vi "Master_CAN.vi"(8 "error in":errorcluster) -> (0 "error out":errorcluster)   [LabVIEW 2018]
uses:
  Type_Def/Type_Def Actuator Controls.ctl
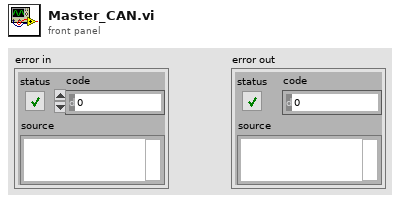
[diagram p1: front panel]
types:
  T1 = typedef "Type_Def Actuator Controls.ctl" = cluster{"Reverse ":bool, "Precharge Ctrl":bool, "Pump Ctrl":bool, "24 VDC Ctr":bool, "Vent Solenoid":bool, "Brake Solenoid":bool, "EMCY  Brake Solenoid":bool, "Digital Out 7B ":bool, "Forward Ctrl":bool, "Contact H1":bool, "Contact L1":bool, "Contact H2":bool, "Contact L2 ":bool, "LED RED":bool, "LED GREEN":bool, " Digital Out 7A":bool}
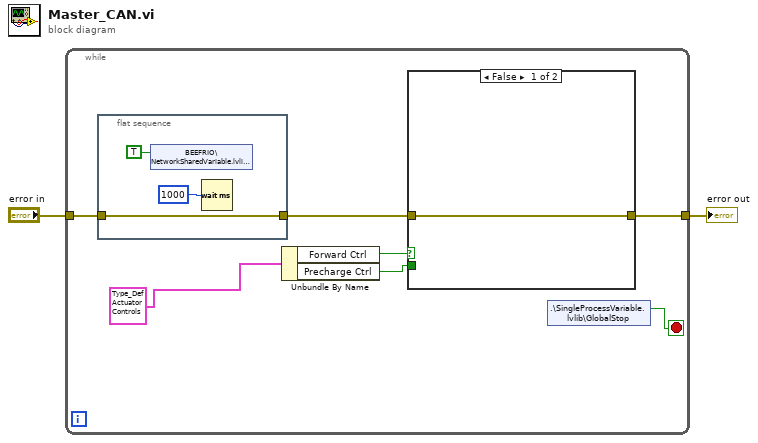
[diagram p0: block diagram]
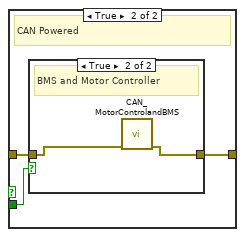
[diagram p2: hidden frame]
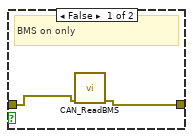
[diagram p3: hidden frame]
diagram:
  n1 = while {
    tunnel: "error in" -> [w8]
    tunnel: [w9] -> w1
    stop <- w6 stop-if-true
    n2 = flat-sequence {
      tunnel: [w19] -> w7
      tunnel: w8 -> [w19]
      frame #0 {
        n3 = shared-variable "BEEFRIO\\NetworkSharedVariable.lvlib\\BMSFreeze"(TRUE ("BMSFreeze")) -> ()  [unwired: 1 in, 1 out]
        n4 = Wait (ms)(milliseconds to wait=u32 1000) -> ()  [unwired: 1 out]
      }
    }
    n5 = Unbundle By Name(T1 {"Reverse "=TRUE, "Precharge Ctrl"=TRUE, "Pump Ctrl"=TRUE, "24 VDC Ctr"=TRUE, "Vent Solenoid"=TRUE, "Brake Solenoid"=TRUE, "EMCY  Brake Solenoid"=TRUE, "Digital Out 7B "=TRUE, "Forward Ctrl"=TRUE, "Contact H1"=TRUE, "Contact L1"=TRUE, "Contact H2"=TRUE, "Contact L2 "=TRUE, "LED RED"=TRUE, "LED GREEN"=TRUE, " Digital Out 7A"=TRUE} ("input cluster")) -> ("Forward Ctrl"=w5:bool, "Precharge Ctrl"=w4:bool)
    n6 = case shown="False" w5 {
      tunnel: [w10 w13] -> w9
      tunnel: w7 -> [w10 w12]
      tunnel: w4 -> [_ w11]
      frame False {
      }
      frame True {
        # "CAN Powered"
        n7 = case shown="True" w11 {
          tunnel: [w14 w16] -> w13
          tunnel: w12 -> [w15 w17]
          frame False {
            # "BMS on only"
            n8 = call "CAN_ReadBMS.vi"("error in (no error)"=w15) -> ("error out"=w14:errorcluster)  [unwired: 10 in]
          }
          frame True {
            # "BMS and Motor Controller"
            n9 = call "CAN_MotorControlandBMS.vi"("error in (no error)"=w17) -> ("error out"=w16:errorcluster)  [unwired: 10 in]
          }
        }
      }
    }
    n10 = shared-variable ".\\SingleProcessVariable.lvlib\\GlobalStop"() -> (w6:bool)  [unwired: 1 in, 1 out]
  }
  "error out" <- w1
